vi "XYRamps [setps.size].vi"(2 "Step size":i32=2000, 3 "Steps":i32=7) -> (0 "Y":dbl[][](graph), 1 "X":dbl[][](graph))   [LabVIEW 2009]
uses:
  <vilib>/Analysis/NI_AALBase.lvlib
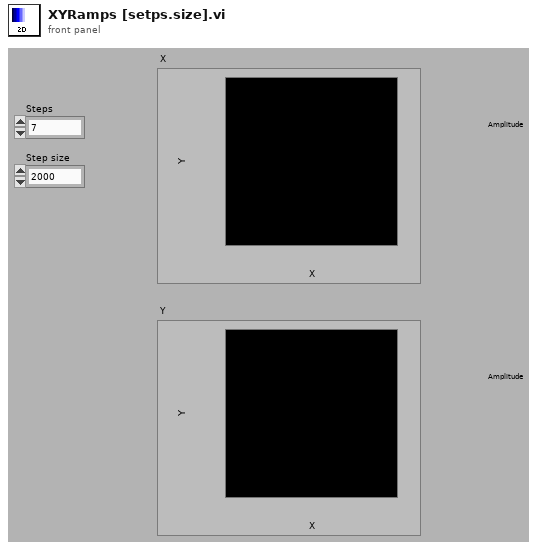
[diagram p1: front panel]
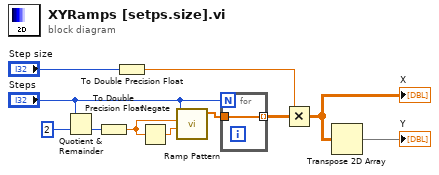
[diagram p0: block diagram]
diagram:
  n1 = Quotient & Remainder(x="Steps", y=2) -> (floor(x/y)=w7:i32)  [unwired: 1 out]
  n2 = To Double Precision Float(number=w7) -> (double precision float=w6:dbl)
  n3 = To Double Precision Float(number="Step size") -> (double precision float=w3:dbl)
  n4 = Negate(x=w6) -> (-x=w11:dbl)
  n5 = call <vilib>:"Ramp Pattern.vi"("start"=w11, "end"=w6, "samples"="Steps") -> ("Ramp Pattern"=w10:dbl[])  [unwired: 2 in, 6 out]
  n6 = for {
    N: "Steps" -> [_]
    tunnel: w10 -> [w12]
    tunnel: [w12] -> w5 mode=indexing
  }
  n7 = Multiply(x=w3, y=w5) -> (x*y=w2:dbl[][])
  "X" <- w2
  n8 = Transpose 2D Array(2D array=w2) -> (transposed array=→"Y":dbl[][])
